vi "Refresh Values.vi"(8 "error in (no error)":errorcluster, 11 "Dynamic Combobox in":refnum<class "Dynamic Combobox.lvclass">) -> (0 "error out":errorcluster, 3 "Dynamic Combobox out":refnum<class "Dynamic Combobox.lvclass">)   [LabVIEW 2020, in "Dynamic Combobox.lvlib" / "Dynamic Combobox.lvclass"]
uses:
  Dynamic Combobox.lvclass
  Dynamic Combobox.lvclass/Dynamic Combobox.ctl
  Dynamic Values/Dynamic Values.lvclass
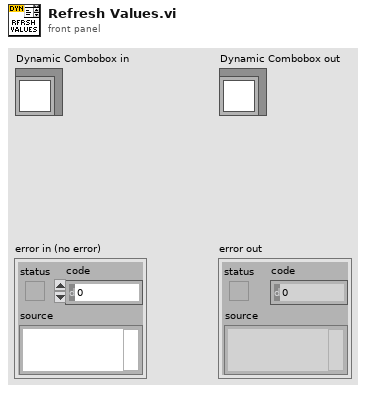
[diagram p1: front panel]
types:
  T1 = typedef "Dynamic Combobox.lvlib/Dynamic Combobox.lvclass/Ref Data.ctl" = cluster{"Values":refnum<class "Dynamic Values.lvclass">, "Debug":bool, "Strings And Values []":T2, "Options":T3}
  T2 = typedef "LVComboBoxStrsAndValuesArrayTypeDef.ctl" = cluster{"String":string, "Value":string}[]
  T3 = typedef "Dynamic Combobox.lvlib/Dynamic Combobox.lvclass/Options.ctl" = cluster{"Browse Entry":bool, "Refresh Entry":bool, "Allow Undefined Values":bool}
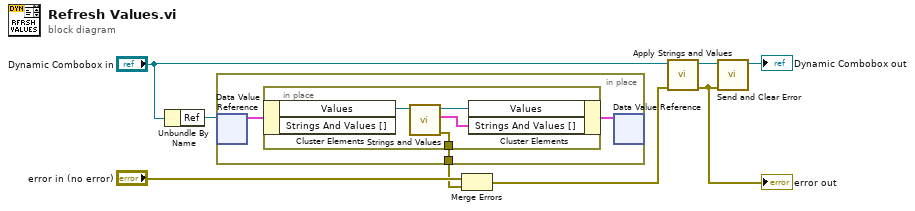
[diagram p0: block diagram]
diagram:
  n1 = Unbundle By Name("Dynamic Combobox in") -> ("Ref"=w6:refnum<data-value>)
  n2 = in-place {
    in-place-border: [w9] -> w4
    n3 = in-place-dvr #1(w6) -> (w11:T1)  [unwired: 1 out]
    n4 = in-place {
      in-place-border: [w13] -> w9
      n5 = in-place-cluster #2(w11) -> ("Values"=w15:refnum<class "Dynamic Values.lvclass">)  [unwired: 1 out]
      n6 = call-dynamic "Strings and Values.vi"("Dynamic Values in"=w15) -> ("error out"=w13:errorcluster, "Strings And Values []"=w12:T2, "Dynamic Values out"=w14:refnum<class "Dynamic Values.lvclass">)  [unwired: 8 in]
      n7 = in-place-cluster #2("Values"=w14, "Strings And Values []"=w12) -> (w10:T1)
    }
    n8 = in-place-dvr #1(w10) -> ()  [unwired: 2 out]
  }
  n9 = Merge Errors("error in (no error)", w4) -> (w7:errorcluster)
  n10 = call "Apply Strings and Values.vi"("error in (no error)"=w7, "Dynamic Combobox in"="Dynamic Combobox in") -> ("error out"=w8:errorcluster, "Dynamic Combobox out"=w1:refnum<class "Dynamic Combobox.lvclass">)  [unwired: 8 in]
  "error out" <- w8
  n11 = call "Send and Clear Error.vi"("error in (no error)"=w8, "Dynamic Combobox in"=w1) -> ("Dynamic Combobox out"=→"Dynamic Combobox out":refnum<class "Dynamic Combobox.lvclass">)  [unwired: 8 in, 1 out]
